vi "20220606-InterpolateCalibration.vi"() -> ()   [LabVIEW 2016]
uses:
  <vilib>/Utility/file.llb/Read Delimited Spreadsheet (DBL).vi
  <vilib>/Utility/file.llb/Write Delimited Spreadsheet (DBL).vi
panel:
  in  "Tab Control":enum32{"讀取檔案", "計算結果"}(tab)=enum."計算結果"
  out "X1(b)":dbl=10.640665
  out "Y1(b)":dbl=769.591376
  out "X2(b)":dbl=390.664468
  out "Y2(b)":dbl=769.591258
  out "X3 (b)":dbl=390.646567
  out "Y3 (b)":dbl=1149.621638
  out "X4 (b)":dbl=10.623763
  out "Y4 (b)":dbl=1149.646079
  out "NOW1":dbl[][](array[numeric])=[[10.640665, 769.591383, 65.509351, -4.3e-05], [390.666052, 769.593118, 65.709351, -4.2e-05], [390.795671, 1149.618756, 65.859351, -4.2e-05], [10.772183, 1149.639611, 65.859351, -4.3e-05]]
  out "NOW2":dbl[][](array[numeric])=[[10.640665, 769.591376, 65.509347, -4.2e-05], [390.664468, 769.591258, 65.759346, -4.2e-05], [390.646567, 1149.621638, 65.809344, -4.2e-05], [10.623763, 1149.646079, 65.859346, -4.2e-05]]
  out "Y2   (a)":dbl=769.593118
  out "X2  (a)":dbl=390.666052
  out "Y1   (a)":dbl=769.591383
  out "X1  (a)":dbl=10.640665
  out "X3(a)":dbl=390.795671
  out "Y3 (a)":dbl=1149.618756
  out "X4 (a)":dbl=10.772183
  out "Y4(a)":dbl=1149.639611
  out "X1":dbl
  out "Y1":dbl=-6.999999982326699e-06
  out "X2":dbl=-0.0015839999999798238
  out "X3":dbl=-0.14910400000002255
  out "X4":dbl=-0.14841999999999977
  out "Y2":dbl=-0.0018599999999651118
  out "Y4":dbl=0.0064680000000407745
  out "Y3":dbl=0.002881999999999607
  in  "目標位址座標":path=path "D:/Gantry_General/Main/ms_kao/gantry path/path data/20220606/c03/C03-1/1 gantry20220606-173814.748.txt"
  in  "目前位址座標":path=path "D:/Gantry_General/Main/ms_kao/gantry path/path data/20220606/c03/C03-1/2 gantry20220606-174010.713.txt"
  out "X1":dbl
  out "Y1":dbl=6.999561588732457e-06
  out "X3":dbl=-0.14909505429676473
  out "Y3":dbl=-0.0028818270903741847
  out "Y2 2":dbl=0.0018598512118681624
  out "X2":dbl=-0.0015838732901166145
  out "X4":dbl=-0.14839863840652387
  out "Y4":dbl=-0.006467069082464956
  out "12*4 2":dbl[][](array[numeric])=[[0.0, 0.0, 0.0, 0.0, 0.0, 0.0, 0.0, 0.0, 0.0, 0.0, 0.0, 0.0], [0.0, 0.0, 0.0, 0.0, 6.999561588732457e-06, 6.999561588732457e-06, -0.0015838732901166145, 0.0018598512118681624, 0.0018598512118681624, 0.0, 0.0, 0.0], [0.0, 0.0, 0.0, -0.14839863840652387, -0.006467069082464956, -0.006467069082464956, -0.14909505429676473, -0.0028818270903741847, -0.0028818270903741847, 0.0, 0.0, 0.0], [0.0, 0.0, 0.0, 0.0, 0.0, 0.0, 0.0, 0.0, 0.0, 0.0, 0.0, 0.0]]
  out "subarray":dbl[][](array[numeric])=[[0.0, 6.999561588732457e-06, 6.999561588732457e-06, -0.0015838732901166145, 0.0018598512118681624, 0.0018598512118681624], [-0.14839863840652387, -0.006467069082464956, -0.006467069082464956, -0.14909505429676473, -0.0028818270903741847, -0.0028818270903741847]]
  in  "需存取的檔案路徑":path=path "D:/Gantry_General/Main/ms_kao/gantry path/path data/20220606/c03/C03-1/c03-1.txt"
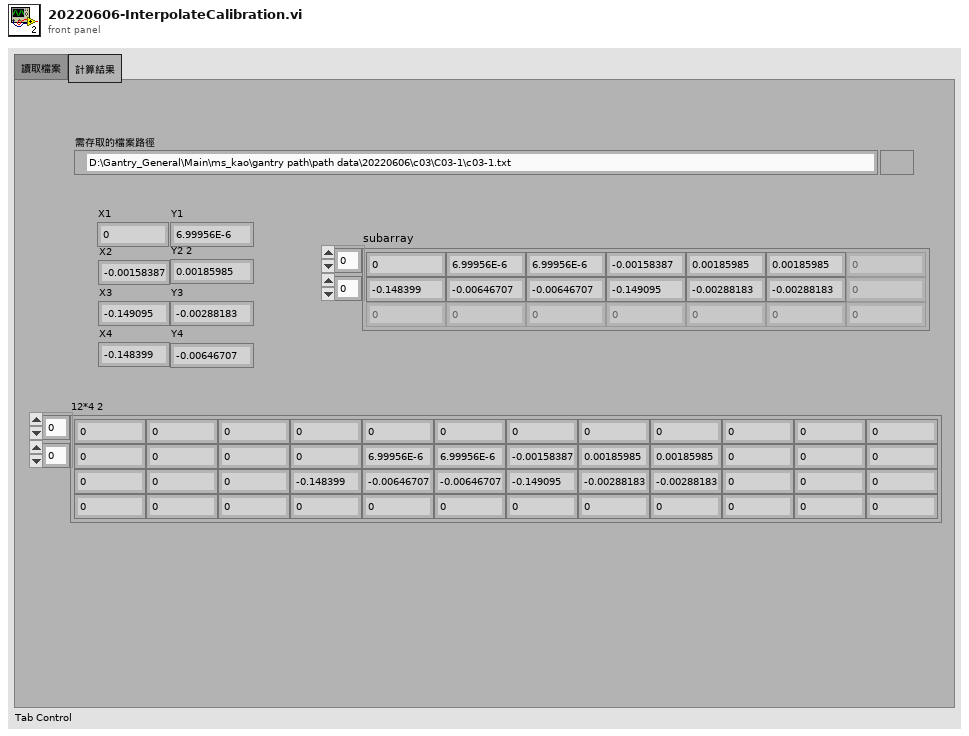
[diagram p1: front panel]
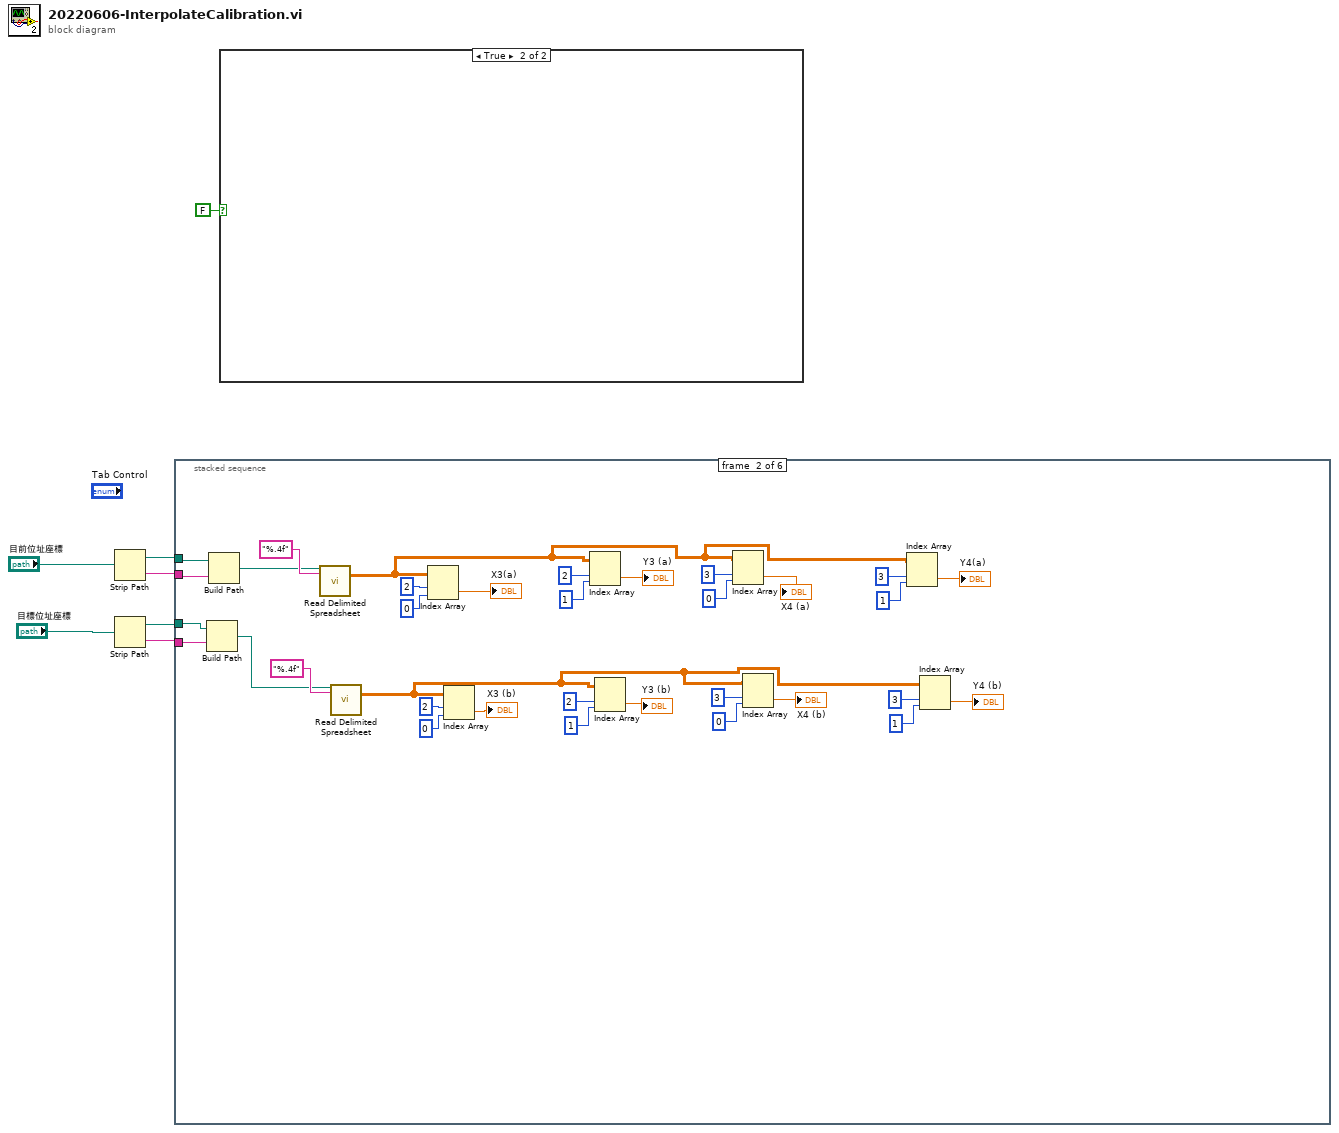
[diagram p0: block diagram]
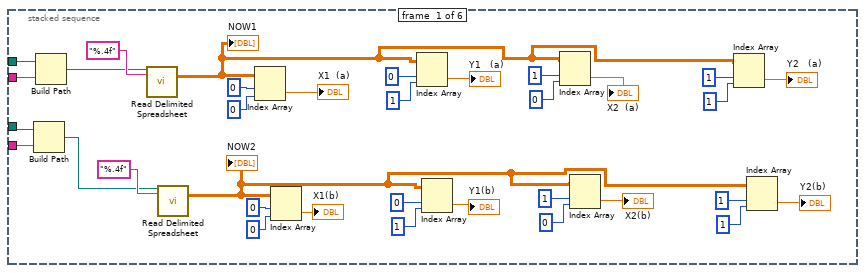
[diagram p3: hidden frame]
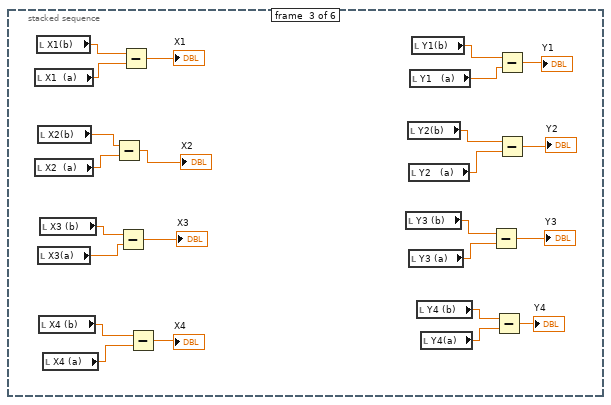
[diagram p4: hidden frame]
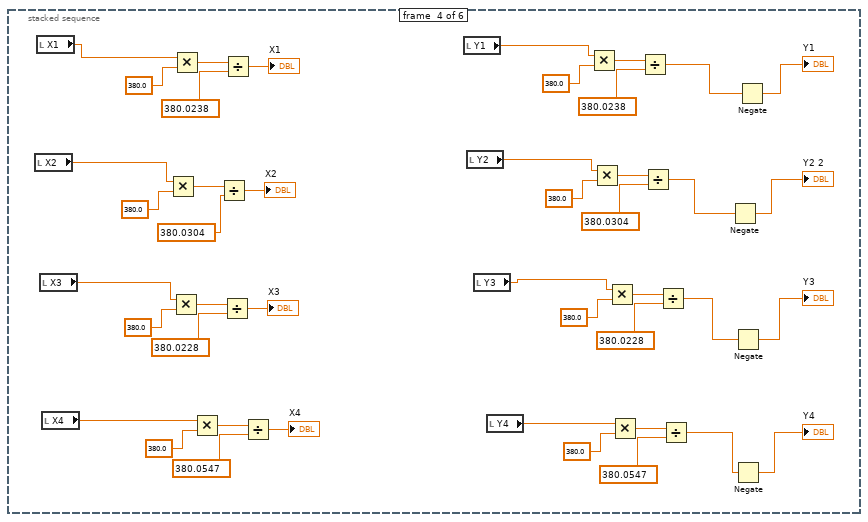
[diagram p5: hidden frame]
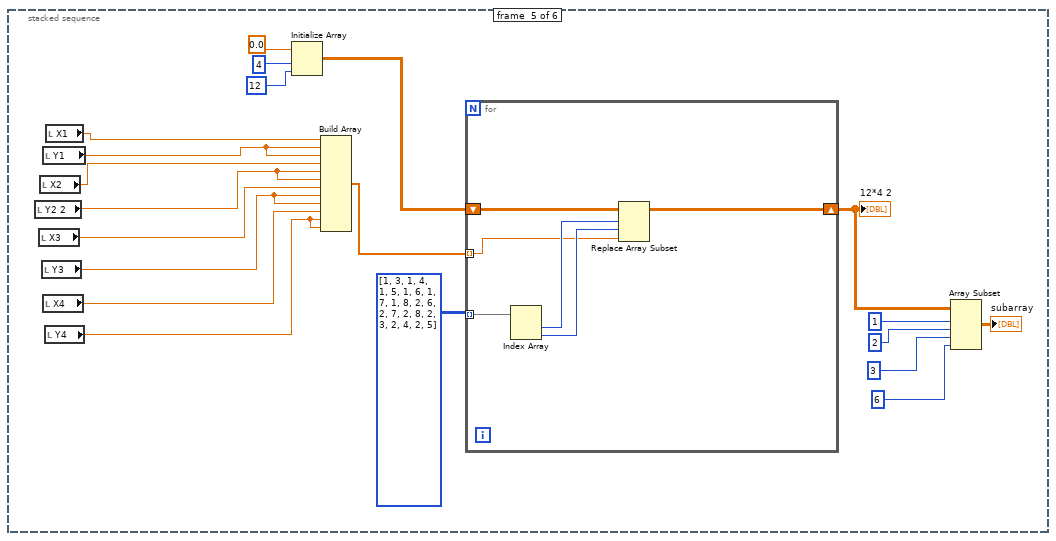
[diagram p6: hidden frame]
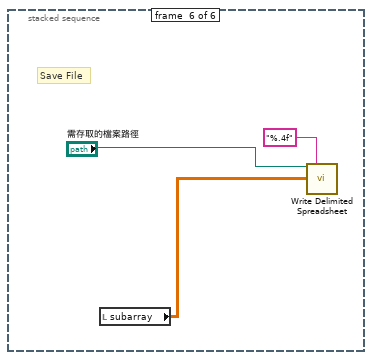
[diagram p7: hidden frame]
diagram:
  n1 = Strip Path(path="目前位址座標") -> (stripped path=w7:path, name=w6:string)
  n2 = Strip Path(path="目標位址座標") -> (stripped path=w5:path, name=w4:string)
  n3 = stacked-sequence {
    tunnel: w7 -> [w37 w42 _ _ _ _]
    tunnel: w6 -> [w35 w43 _ _ _ _]
    tunnel: w5 -> [w34 w44 _ _ _ _]
    tunnel: w4 -> [w33 w45 _ _ _ _]
    frame #0 {
      n4 = Build Path(base path=w34, name or relative path=w33) -> (appended path=w28:path)
      n5 = Build Path(base path=w37, name or relative path=w35) -> (appended path=w36:path)
      n6 = call-poly <vilib>:"Read Delimited Spreadsheet.vi"("file path (dialog if empty)"=w36, "format (%.3f)"="%.4f") -> ("all rows"=w8:dbl[][])  [unwired: 8 in, 5 out]
      "NOW1" <- w8
      n7 = call-poly <vilib>:"Read Delimited Spreadsheet.vi"("file path (dialog if empty)"=w28, "format (%.3f)"="%.4f") -> ("all rows"=w12:dbl[][])  [unwired: 8 in, 5 out]
      "NOW2" <- w12
      n8 = Index Array(array=w8, index (row)=0, index (col)=0 ("disabled index (col)")) -> (element=→"X1  (a)":dbl)
      n9 = Index Array(array=w12, index (row)=0, index (col)=0 ("disabled index (col)")) -> (element=→"X1(b)":dbl)
      n10 = Index Array(array=w8, index (row)=0, index (col)=1 ("disabled index (col)")) -> (element=→"Y1   (a)":dbl)
      n11 = Index Array(array=w12, index (row)=0, index (col)=1 ("disabled index (col)")) -> (element=→"Y1(b)":dbl)
      n12 = Index Array(array=w8, index (row)=1, index (col)=0 ("disabled index (col)")) -> (element=→"X2  (a)":dbl)
      n13 = Index Array(array=w12, index (row)=1, index (col)=0 ("disabled index (col)")) -> (element=→"X2(b)":dbl)
      n14 = Index Array(array=w8, index (row)=1, index (col)=1 ("disabled index (col)")) -> (element=→"Y2   (a)":dbl)
      n15 = Index Array(array=w12, index (row)=1, index (col)=1 ("disabled index (col)")) -> (element=→"Y2(b)":dbl)
    }
    frame #1 {
      n16 = Build Path(base path=w44, name or relative path=w45) -> (appended path=w66:path)
      n17 = Build Path(base path=w42, name or relative path=w43) -> (appended path=w71:path)
      n18 = call-poly <vilib>:"Read Delimited Spreadsheet.vi"("file path (dialog if empty)"=w71, "format (%.3f)"="%.4f") -> ("all rows"=w46:dbl[][])  [unwired: 8 in, 5 out]
      n19 = call-poly <vilib>:"Read Delimited Spreadsheet.vi"("file path (dialog if empty)"=w66, "format (%.3f)"="%.4f") -> ("all rows"=w50:dbl[][])  [unwired: 8 in, 5 out]
      n20 = Index Array(array=w46, index (row)=2, index (col)=0 ("disabled index (col)")) -> (element=→"X3(a)":dbl)
      n21 = Index Array(array=w50, index (row)=2, index (col)=0 ("disabled index (col)")) -> (element=→"X3 (b)":dbl)
      n22 = Index Array(array=w46, index (row)=2, index (col)=1 ("disabled index (col)")) -> (element=→"Y3 (a)":dbl)
      n23 = Index Array(array=w50, index (row)=2, index (col)=1 ("disabled index (col)")) -> (element=→"Y3 (b)":dbl)
      n24 = Index Array(array=w46, index (row)=3, index (col)=0 ("disabled index (col)")) -> (element=→"X4 (a)":dbl)
      n25 = Index Array(array=w50, index (row)=3, index (col)=0 ("disabled index (col)")) -> (element=→"X4 (b)":dbl)
      n26 = Index Array(array=w46, index (row)=3, index (col)=1 ("disabled index (col)")) -> (element=→"Y4(a)":dbl)
      n27 = Index Array(array=w50, index (row)=3, index (col)=1 ("disabled index (col)")) -> (element=→"Y4 (b)":dbl)
    }
    frame #2 {
      n28 = local read "X1  (a)"() -> (w98:dbl)
      n29 = local read "X2  (a)"() -> (w95:dbl)
      n30 = local read "X1(b)"() -> (w99:dbl)
      n31 = local read "X2(b)"() -> (w94:dbl)
      n32 = local read "X3(a)"() -> (w92:dbl)
      n33 = local read "X4 (b)"() -> (w87:dbl)
      n34 = local read "X3 (b)"() -> (w93:dbl)
      n35 = local read "X4 (a)"() -> (w86:dbl)
      n36 = Subtract(x=w94, y=w95) -> (x-y=→"X2":dbl)
      n37 = Subtract(x=w93, y=w92) -> (x-y=→"X3":dbl)
      n38 = Subtract(x=w99, y=w98) -> (x-y=→"X1":dbl)
      n39 = Subtract(x=w87, y=w86) -> (x-y=→"X4":dbl)
      n40 = local read "Y3 (b)"() -> (w89:dbl)
      n41 = local read "Y2(b)"() -> (w85:dbl)
      n42 = local read "Y2   (a)"() -> (w84:dbl)
      n43 = local read "Y3 (a)"() -> (w88:dbl)
      n44 = local read "Y1   (a)"() -> (w96:dbl)
      n45 = local read "Y1(b)"() -> (w97:dbl)
      n46 = local read "Y4 (b)"() -> (w91:dbl)
      n47 = local read "Y4(a)"() -> (w90:dbl)
      n48 = Subtract(x=w89, y=w88) -> (x-y=→"Y3":dbl)
      n49 = Subtract(x=w91, y=w90) -> (x-y=→"Y4":dbl)
      n50 = Subtract(x=w97, y=w96) -> (x-y=→"Y1":dbl)
      n51 = Subtract(x=w85, y=w84) -> (x-y=→"Y2":dbl)
    }
    frame #3 {
      n52 = local read "X2"() -> (w114:dbl)
      n53 = local read "X1"() -> (w115:dbl)
      n54 = local read "X3"() -> (w110:dbl)
      n55 = local read "X4"() -> (w109:dbl)
      n56 = Multiply(x=w114, y=380.0) -> (x*y=w130:dbl)
      n57 = Multiply(x=w110, y=380.0) -> (x*y=w128:dbl)
      n58 = Multiply(x=w115, y=380.0) -> (x*y=w133:dbl)
      n59 = Multiply(x=w109, y=380.0) -> (x*y=w124:dbl)
      n60 = Divide(x=w130, y=380.0304) -> (x/y=→"X2":dbl)
      n61 = Divide(x=w128, y=380.0228) -> (x/y=→"X3":dbl)
      n62 = Divide(x=w133, y=380.0238) -> (x/y=→"X1":dbl)
      n63 = Divide(x=w124, y=380.0547) -> (x/y=→"X4":dbl)
      n64 = local read "Y1"() -> (w113:dbl)
      n65 = local read "Y2"() -> (w112:dbl)
      n66 = local read "Y3"() -> (w111:dbl)
      n67 = local read "Y4"() -> (w108:dbl)
      n68 = Multiply(x=w113, y=380.0) -> (x*y=w142:dbl)
      n69 = Multiply(x=w112, y=380.0) -> (x*y=w139:dbl)
      n70 = Multiply(x=w111, y=380.0) -> (x*y=w136:dbl)
      n71 = Multiply(x=w108, y=380.0) -> (x*y=w121:dbl)
      n72 = Divide(x=w142, y=380.0238) -> (x/y=w107:dbl)
      n73 = Divide(x=w139, y=380.0304) -> (x/y=w101:dbl)
      n74 = Divide(x=w136, y=380.0228) -> (x/y=w103:dbl)
      n75 = Divide(x=w121, y=380.0547) -> (x/y=w105:dbl)
      n76 = Negate(x=w101) -> (-x=→"Y2 2":dbl)
      n77 = Negate(x=w103) -> (-x=→"Y3":dbl)
      n78 = Negate(x=w105) -> (-x=→"Y4":dbl)
      n79 = Negate(x=w107) -> (-x=→"Y1":dbl)
    }
    frame #4 {
      n80 = local read "Y2 2"() -> (w157:dbl)
      n81 = local read "X3"() -> (w156:dbl)
      n82 = local read "X2"() -> (w158:dbl)
      n83 = local read "Y3"() -> (w155:dbl)
      n84 = local read "Y1"() -> (w159:dbl)
      n85 = local read "X4"() -> (w154:dbl)
      n86 = local read "Y4"() -> (w153:dbl)
      n87 = local read "X1"() -> (w160:dbl)
      n88 = Initialize Array(0.0 ("element"), 4 ("dimension size"), 12 ("dimension size")) -> (w150:dbl[][])
      n89 = Build Array(w160, w159, w159, w158, w157, w157, w156, w155, w155, w154, w153, w153) -> (w152:dbl[])
      n90 = for {
        tunnel: w152 -> [w165] mode=indexing
        tunnel: i32[][] [[1, 3], [1, 4], [1, 5], [1, 6], [1, 7], [1, 8], [2, 6], [2, 7], [2, 8], [2, 3], [2, 4], [2, 5]] -> [w169] mode=indexing
        shift-right: [w164] -> w149
        shift-left: w150 -> [w168]
        n91 = Index Array "Index Array"(array=w169) -> (element #1=w167:i32, element #2=w166:i32)  [unwired: 2 in]
        n92 = Replace Array Subset "Replace Array Subset"(array=w168, new element=w165, index (row)=w167, index (col)=w166) -> (w164:dbl[][])
      }
      "12*4 2" <- w149
      n93 = Array Subset(array=w149, index (row)=1 ("index"), length (row)=2 ("index"), index (col)=3 ("index"), length (col)=6 ("index")) -> (→"subarray":dbl[][])
    }
    frame #5 {
      # "Save File"
      n94 = local read "subarray"() -> (w172:dbl[][])
      n95 = call-poly <vilib>:"Write Delimited Spreadsheet.vi"("file path (dialog if empty)"="需存取的檔案路徑", "format (%.3f)"="%.4f", "2D data"=w172) -> ()  [unwired: 11 in, 2 out]
    }
  }
  n96 = case shown="True" FALSE {
    frame False {
    }
    frame True {
    }
  }
